vi "Get VI Description and Help.vi"(10 "VI Index":i32, 11 "VI Data in":T1[](array[typedef])) -> (1 "VI Description":string, 3 "VI Data out":T1[](array[typedef]), 4 "Help Tag":string, 6 "Help Path":string)   [LabVIEW 2023, in "VI Properties Editor.lvlib"]
uses:
  VI Properties Editor.lvlib
  Cluster Data.ctl
  <vilib>/picture/picture.llb/imagedata.ctl
panel:
  # "Connector Pane"
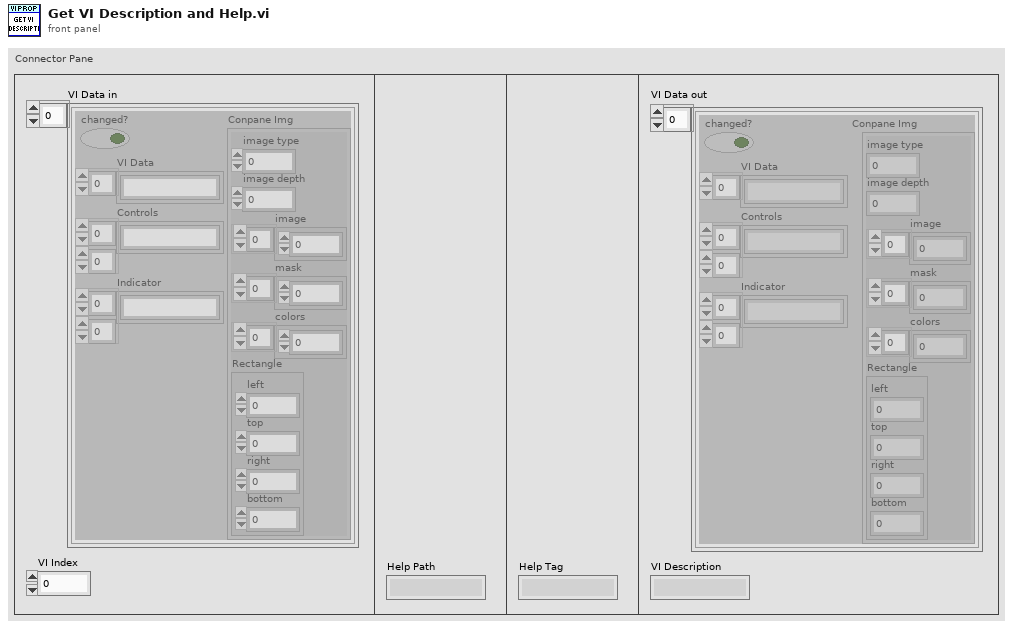
[diagram p1: front panel]
types:
  T1 = typedef "VI Properties Editor.lvlib/Cluster Data.ctl" = cluster{"changed?":bool, "VI Data":string[], "Controls":string[][], "Indicator":string[][], "Conpane Img":T2}
  T2 = typedef "imagedata.ctl" = cluster{"image type":i32, "image depth":i32, "image":u8[], "mask":u8[], "colors":u32[], "Rectangle":cluster{"left":i16, "top":i16, "right":i16, "bottom":i16}}
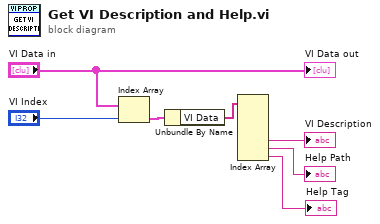
[diagram p0: block diagram]
diagram:
  n1 = Index Array(array="VI Data in", index="VI Index") -> (element=w4:T1)
  n2 = Unbundle By Name(w4) -> ("VI Data"=w7:string[])
  n3 = Index Array(array=w7) -> (element #4=→"VI Description":string, element #5=→"Help Path":string, element #6=→"Help Tag":string)  [unwired: 6 in, 3 out]
  "VI Data out" <- "VI Data in"
